vi "Tabor 5064 - Set Channel Frequency (SubVI).vi"(6 "write_delay (ms)":u32=100, 7 "GPIB Address":string="4", 8 "error_in":errorcluster, 11 "frequency":dbl=41.0 format="%#_13g") -> (0 "error_out":errorcluster)   [LabVIEW 2018]
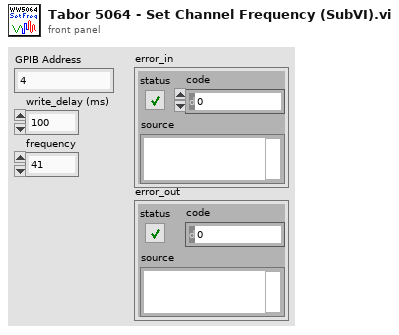
[diagram p1: front panel]
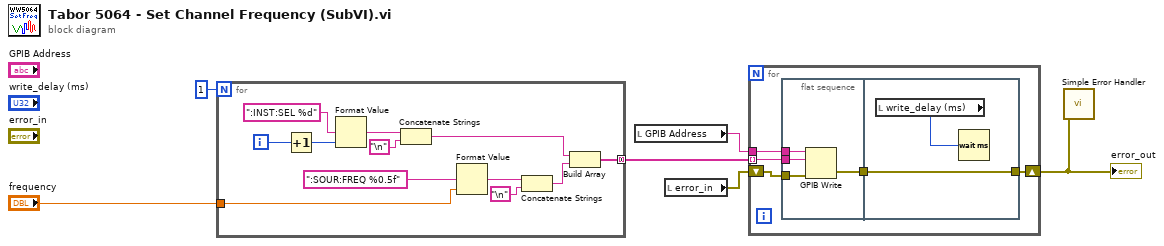
[diagram p0: block diagram]
diagram:
  n1 = for {
    N: 1 -> [_]
    tunnel: [w10] -> w5 mode=concatenating
    tunnel: "frequency" -> [w7]
    i -> [w15]
    n2 = Increment(x=w15) -> (x+1=w16:i32)
    n3 = Format Value(format string=":INST:SEL %d", value (0)=w16) -> (output string=w12:string)  [unwired: 1 in]
    n4 = Concatenate Strings(w12, "\n") -> (w11:string)
    n5 = Format Value(format string=":SOUR:FREQ %0.5f", value (0)=w7) -> (output string=w9:string)  [unwired: 1 in]
    n6 = Concatenate Strings(w9, "\n") -> (w8:string)
    n7 = Build Array(w11, w8) -> (w10:string[])
  }
  n8 = local read "GPIB Address"() -> (w4:string)
  n9 = local read "error_in"() -> (w3:errorcluster)
  n10 = for {
    tunnel: w4 -> [w23]
    tunnel: w5 -> [w22] mode=indexing
    shift-right: [w21] -> w6
    shift-left: w3 -> [w20]
    n11 = flat-sequence {
      tunnel: w23 -> [w27]
      tunnel: w22 -> [w26]
      tunnel: w20 -> [w24]
      tunnel: [w25] -> w19
      tunnel: [w29] -> w21
      tunnel: w19 -> [w29]
      frame #0 {
        n12 = GPIB Write(0:w27, 1:w26, 3:w24) -> (6:w25:errorcluster)  [unwired: 2 in, 1 out]
      }
      frame #1 {
        n13 = local read "write_delay (ms)"() -> (w28:u32)
        n14 = Wait (ms)(milliseconds to wait=w28) -> ()  [unwired: 1 out]
      }
    }
  }
  "error_out" <- w6
  n15 = call <vilib>:"Simple Error Handler.vi"("error in (no error)"=w6) -> ()  [unwired: 4 in, 5 out]
